vi "Do Core.vi"(8 "error in":errorcluster, 9 "Actor in":refnum<class "Actor.lvclass">, 11 "Reply Msg DS in":refnum<class "Reply Msg DataSocket Msg.lvclass">) -> (0 "error out":errorcluster, 1 "Actor out":refnum<class "Actor.lvclass">, 2 "Reply":variant)   [LabVIEW 2023, in "Target Reply Time Test Actor.lvlib" / "Reply Msg DataSocket Msg.lvclass"]
uses:
  Reply Msg DataSocket Msg.lvclass
  <vilib>/ActorFramework/Actor/Actor.lvclass
  Target Reply Time Test Actor/Target Reply Time Test Actor.lvclass
  C:/Program Files/National Instruments/LabVIEW 2023/vi.lib/ActorFramework/Actor/Actor.lvclass
  Reply Msg DataSocket Msg.lvclass/Reply Msg DataSocket Msg.ctl
  9ce2371d-5a1b-4ae0-b52b-723504647e81.vi
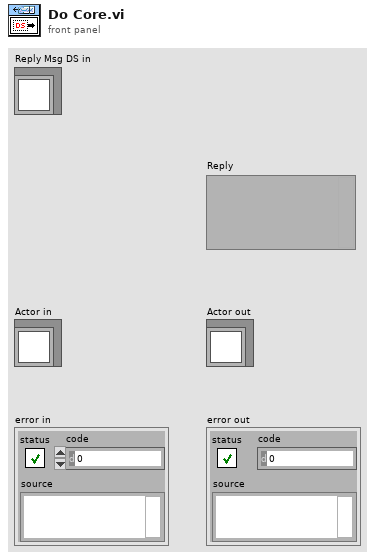
[diagram p1: front panel]
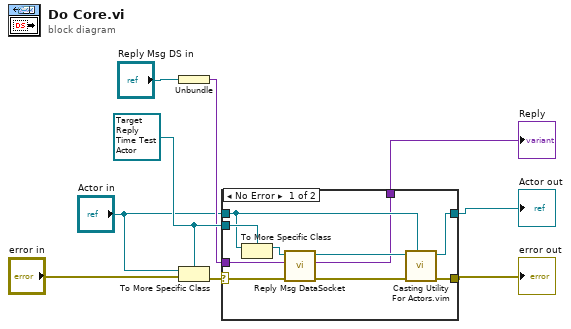
[diagram p0: block diagram]
diagram:
  w8 = refnum<class "Target Reply Time Test Actor.lvclass"> refnum ("Actor in")
  n1 = Unbundle("Reply Msg DS in") -> (w7:variant)
  n2 = To More Specific Class(target class=w8, reference="Actor in", error in="error in") -> (error out=w9:errorcluster)  [unwired: 1 out]
  n3 = case shown="No Error" w9 {
    selector: w9 -> [w19 w21]
    tunnel: [w13 w21] -> w6
    tunnel: [w14 w20] -> w5
    tunnel: "Actor in" -> [w16 w20]
    tunnel: w8 -> [w17 _]
    tunnel: w7 -> [w11 _]
    tunnel: [w10 _] -> w4
    frame No Error {
      n4 = To More Specific Class(target class=w17, reference=w16) -> (specific class reference=w18:refnum<class "Target Reply Time Test Actor.lvclass">)  [unwired: 1 in, 1 out]
      n5 = call-dynamic "Reply Msg DataSocket.vi"("error in (no error)"=w19, "Input"=w11, "Target Reply Time Test Actor in"=w18) -> ("error out"=w12:errorcluster, "Output"=w10:variant, "Target Reply Time Test Actor out"=w15:refnum<class "Target Reply Time Test Actor.lvclass">)  [unwired: 6 in]
      n6 = call "Casting Utility For Actors.vim"("type"=w16, "error in (no error)"=w12, "Actor in"=w15) -> ("error out"=w13:errorcluster, "Actor out"=w14:refnum<class "Actor.lvclass">)  [unwired: 7 in]
    }
    frame Error {
      # "If type check fails, pass the original object out again."
    }
  }
  "error out" <- w6
  "Actor out" <- w5
  "Reply" <- w4
